vi "PPR_TRAJECTORY_GLOBALS.vi"() -> ()   [LabVIEW 2019]
uses:
  <vilib>/Rock Robotics/WPI/ThirdParty/JAS_Junk/TrajLib/TypeDef/POSE2D.ctl
  <vilib>/Rock Robotics/WPI/ThirdParty/JAS_Junk/TrajLib/TypeDef/TRANSLATION2D.ctl
  <vilib>/Rock Robotics/WPI/ThirdParty/JAS_Junk/TrajLib/TypeDef/ROTATION2D.ctl
  <vilib>/Rock Robotics/WPI/ThirdParty/MJansen/PathPlanner/TypeDef/PathPlannerTrajectory.ctl
  <vilib>/Rock Robotics/WPI/ThirdParty/MJansen/PathPlanner/TypeDef/PathPlannerTrajectoryState.ctl
  <vilib>/Rock Robotics/WPI/ThirdParty/MJansen/PathPlanner/TypeDef/PathPlannerPathConstraints.ctl
  <vilib>/Rock Robotics/WPI/ThirdParty/JAS_Junk/TrajLib/TypeDef/DIFF_DRIVE_ODOM2.ctl
  <vilib>/Rock Robotics/WPI/ThirdParty/JAS_Junk/TrajLib/Trajectory_Library.lvlib
  <vilib>/Rock Robotics/WPI/ThirdParty/MJansen/PathPlanner/PathPlanner24.lvlib
panel:
  out "Traj Pos Error FT":dbl format="%17.2f"
  in  "Absolute Trajectory":T1 {"States"."TargetHolonomicRotation"."SIN" format="%13.4f"; "States"."TargetHolonomicRotation"."COS" format="%13.4f"; "States"."TargetHolonomicRotation"."VALUE" format="%13.4f"; "States"."Heading"."SIN" format="%13.4f"; "States"."Heading"."COS" format="%13.4f"; "States"."Heading"."VALUE" format="%13.4f"; "States"."PositionMeters"."Y" format="%14.3f"; "States"."PositionMeters"."X" format="%14.3f"}
  out "Other ABS Odom Pose":T6={"TRANSLATION"={"X"=0.0, "Y"=0.0}, "ROTATION"={"VALUE"=0.0, "COS"=1.0, "SIN"=0.0}} {"ROTATION"."SIN" format="%13.4f"; "ROTATION"."COS" format="%13.4f"; "ROTATION"."VALUE" format="%13.4f"; "TRANSLATION"."Y" format="%14.3f"; "TRANSLATION"."X" format="%14.3f"}
  out "Current Trajectory State":T2={"TimeSeconds"=0.0, "VelocityMPS"=0.0, "AccerationMpsSq"=0.0, "HeadingAngularVelRadPerSec"=0.0, "PositionMeters"={"X"=0.0, "Y"=0.0}, "Heading"={"VALUE"=0.0, "COS"=1.0, "SIN"=0.0}, "TargetHolonomicRotation"={"VALUE"=0.0, "COS"=1.0, "SIN"=0.0}, "CurvatureRadPerMeter"=0.0, "PathPlannerConstraints"={"MaxVelocityMps;"=0.0, "MaxAccelerationMpsSq;"=0.0, "MaxAngularVelRadPsEc;"=0.0, "MaxAngularAccRadPSecSq"=0.0, "Exists"=FALSE, "Unlimited"=FALSE, "NominalVoltageVolts"=12.0}, "DeltaPos"=0.0} {"TargetHolonomicRotation"."SIN" format="%13.4f"; "TargetHolonomicRotation"."COS" format="%13.4f"; "TargetHolonomicRotation"."VALUE" format="%13.4f"; "Heading"."SIN" format="%13.4f"; "Heading"."COS" format="%13.4f"; "Heading"."VALUE" format="%13.4f"; "PositionMeters"."Y" format="%14.3f"; "PositionMeters"."X" format="%14.3f"}
  in  "Initial Absolute Pose":T6 {"ROTATION"."SIN" format="%13.4f"; "ROTATION"."COS" format="%13.4f"; "ROTATION"."VALUE" format="%13.4f"; "TRANSLATION"."Y" format="%14.3f"; "TRANSLATION"."X" format="%14.3f"}
  out "Absolute Odometry Pose":T6={"TRANSLATION"={"X"=0.0, "Y"=0.0}, "ROTATION"={"VALUE"=0.0, "COS"=1.0, "SIN"=0.0}} {"ROTATION"."SIN" format="%13.4f"; "ROTATION"."COS" format="%13.4f"; "ROTATION"."VALUE" format="%13.4f"; "TRANSLATION"."Y" format="%14.3f"; "TRANSLATION"."X" format="%14.3f"}
  out "Absolute Odometry":T7={"M_POSE_Meters"={"TRANSLATION"={"X"=0.0, "Y"=0.0}, "ROTATION"={"VALUE"=0.0, "COS"=1.0, "SIN"=0.0}}, "M_GyroOffset"={"VALUE"=0.0, "COS"=1.0, "SIN"=0.0}, "M_PrevAngle"={"VALUE"=0.0, "COS"=1.0, "SIN"=0.0}, "M_PrevLeftDist_M"=0.0, "M_PrevRightDist_M"=0.0, "M_InitLeftDist_M"=0.0, "M_InitRightDist_M"=0.0} {"M_PrevAngle"."SIN" format="%13.4f"; "M_PrevAngle"."COS" format="%13.4f"; "M_PrevAngle"."VALUE" format="%13.4f"; "M_GyroOffset"."SIN" format="%13.4f"; "M_GyroOffset"."COS" format="%13.4f"; "M_GyroOffset"."VALUE" format="%13.4f"; "M_POSE_Meters"."ROTATION"."SIN" format="%13.4f"; "M_POSE_Meters"."ROTATION"."COS" format="%13.4f"; "M_POSE_Meters"."ROTATION"."VALUE" format="%13.4f"; "M_POSE_Meters"."TRANSLATION"."Y" format="%14.3f"; "M_POSE_Meters"."TRANSLATION"."X" format="%14.3f"}
  in  "Relative_Trajectory":T1 {"States"."TargetHolonomicRotation"."SIN" format="%13.4f"; "States"."TargetHolonomicRotation"."COS" format="%13.4f"; "States"."TargetHolonomicRotation"."VALUE" format="%13.4f"; "States"."Heading"."SIN" format="%13.4f"; "States"."Heading"."COS" format="%13.4f"; "States"."Heading"."VALUE" format="%13.4f"; "States"."PositionMeters"."Y" format="%14.3f"; "States"."PositionMeters"."X" format="%14.3f"}
  out "Traj Rot Vel FF Rad/Sec":dbl format="%17.2f"
  out "Traj_Sample_Time_Sec":dbl format="%17.2f"
  out "Traj Final Heading Dmd Deg":dbl format="%17.2f"
  out "Relative Trajectory Pose":T6={"TRANSLATION"={"X"=0.0, "Y"=0.0}, "ROTATION"={"VALUE"=0.0, "COS"=1.0, "SIN"=0.0}} {"ROTATION"."SIN" format="%13.4f"; "ROTATION"."COS" format="%13.4f"; "ROTATION"."VALUE" format="%13.4f"; "TRANSLATION"."Y" format="%14.3f"; "TRANSLATION"."X" format="%14.3f"}
  out "Traj Heading Dmd Deg":dbl format="%17.2f"
  out "Traj Y Corr":dbl format="%17.2f"
  out "Traj X Corr":dbl format="%17.2f"
  out "Traj Closed Loop":bool
  out "Traj Curvature Sample":dbl format="%17.2f"
  out "Traj Velocity Sample":dbl format="%17.2f"
  out "Traj Heading Sample":dbl format="%17.2f"
  out "Traj Y Sample":dbl format="%17.2f"
  out "Traj X Sample":dbl format="%17.2f"
  out "Traj_IsGood":bool
  out "Traj_Total_Time":dbl format="%17.2f"
  out "Traj_Total_States":dbl format="%17.2f"
  out "Traj Heading Err_DEG":dbl format="%17.2f"
  out "Traj Y Err_FT":dbl format="%17.2f"
  out "Traj X Err_FT":dbl format="%17.2f"
  out "Traj_OnTarget":bool
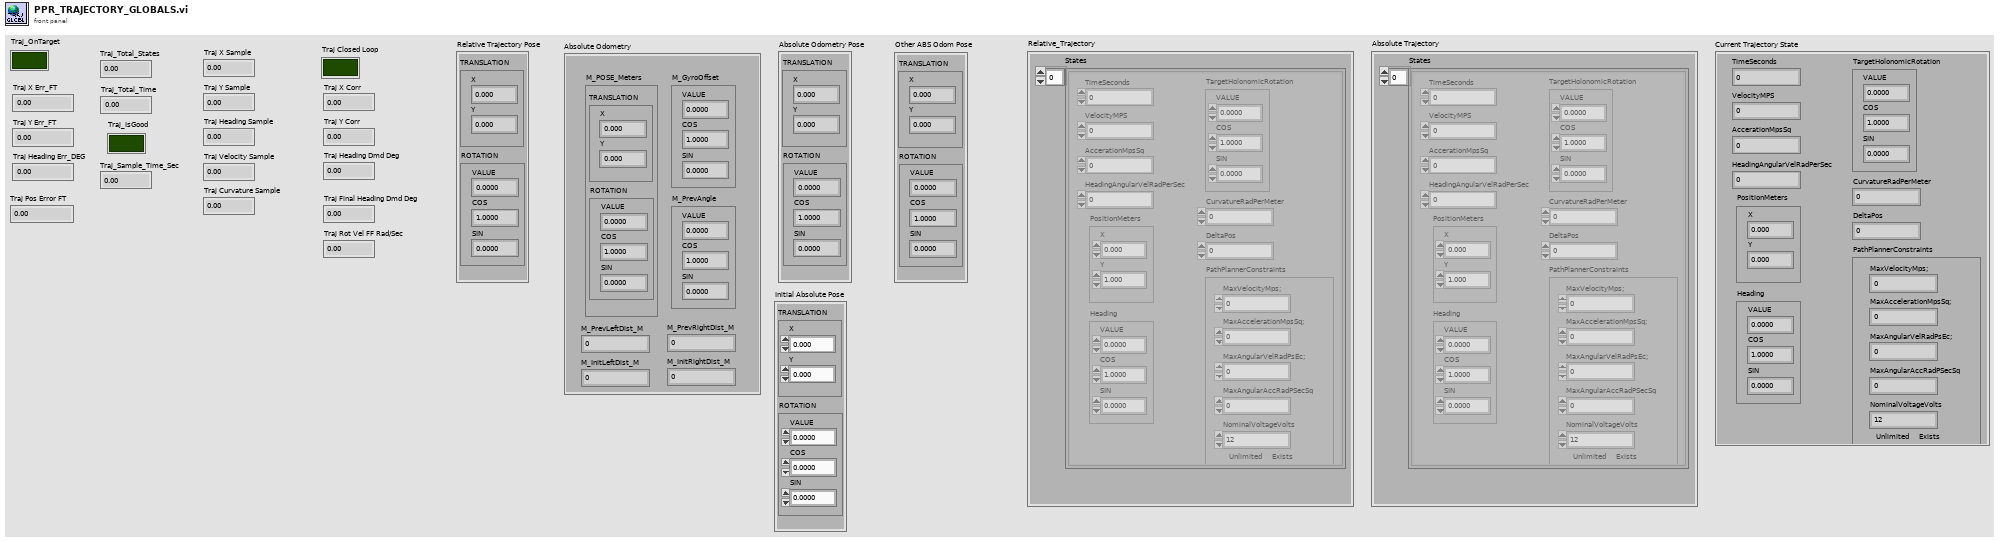
[diagram p1: front panel]
types:
  T1 = typedef "PathPlanner24.lvlib/PathPlannerTrajectory.ctl" = cluster{"States":T2[]}
  T2 = typedef "PathPlanner24.lvlib/PathPlannerTrajectoryState.ctl" = cluster{"TimeSeconds":dbl, "VelocityMPS":dbl, "AccerationMpsSq":dbl, "HeadingAngularVelRadPerSec":dbl, "PositionMeters":T3, "Heading":T4, "TargetHolonomicRotation":T4, "CurvatureRadPerMeter":dbl, "PathPlannerConstraints":T5, "DeltaPos":dbl}
  T3 = typedef "Trajectory_Library.lvlib/TRANSLATION2D.ctl" = cluster{"X":dbl, "Y":dbl}
  T4 = typedef "Trajectory_Library.lvlib/ROTATION2D.ctl" = cluster{"VALUE":dbl, "COS":dbl, "SIN":dbl}
  T5 = typedef "PathPlanner24.lvlib/PathPlannerPathConstraints.ctl" = cluster{"MaxVelocityMps;":dbl, "MaxAccelerationMpsSq;":dbl, "MaxAngularVelRadPsEc;":dbl, "MaxAngularAccRadPSecSq":dbl, "Exists":bool, "Unlimited":bool, "NominalVoltageVolts":dbl}
  T6 = typedef "Trajectory_Library.lvlib/POSE2D.ctl" = cluster{"TRANSLATION":T3, "ROTATION":T4}
  T7 = typedef "Trajectory_Library.lvlib/DIFF_DRIVE_ODOM2.ctl" = cluster{"M_POSE_Meters":T6, "M_GyroOffset":T4, "M_PrevAngle":T4, "M_PrevLeftDist_M":dbl, "M_PrevRightDist_M":dbl, "M_InitLeftDist_M":dbl, "M_InitRightDist_M":dbl}
diagram:
